vi "Send Message And Wait For Response.vi"(7 "Message Priority (Normal)":T1=enum."Normal", 8 "error in (no error)":errorcluster, 9 "timeout in ms (-1)":i32=-1, 10 "Original Message":refnum<class "Reply Msg.lvclass">, 11 "Message Enqueuer in":refnum<class "Message Enqueuer.lvclass">) -> (0 "error out":errorcluster, 1 "timed out?":bool, 2 "Reply":variant, 3 "Message Enqueuer out":refnum<class "Message Enqueuer.lvclass">)   [LabVIEW 2020, in "Reply Msg.lvclass"]
doc: "This message is <b>DEPRECATED</b>. Please replace it with <b>AF Specialty Messages.lvlib:Reply Msg.lvclass</b>, which provides the same functionality and a cleaner PPL build experience.\n\n<p>(<strong>Filename</strong>: <span class=\"dnl\">Actor Framework.lvlib:Reply Msg.lvclass:Send Message And Wait For Response.vi</span>)</p>\n\n<p>Sends a message to an actor and synchronously waits for a response from the actor.</p>"
uses:
  Reply Msg.lvclass
  C:/dev/actor-framework/dist/vi.lib/ActorFramework/Message/Message.lvclass
  Message Enqueuer/Message Enqueuer.lvclass
  Reply Msg.lvclass/Reply Msg.ctl
  Message Enqueuer/Message Enqueuer.lvclass/Message Enqueuer.ctl
  Message Enqueuer/Message Priority.ctl
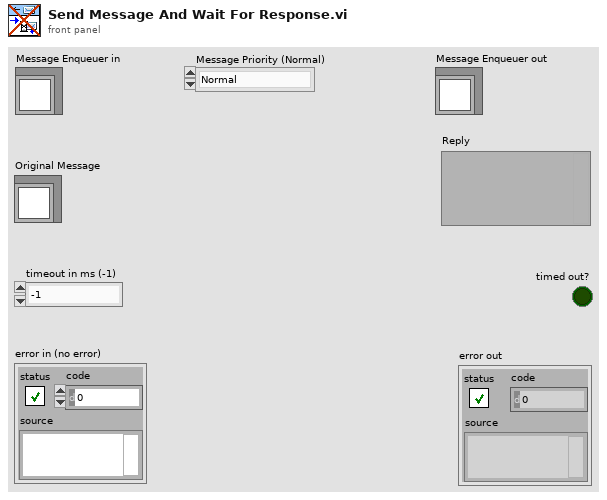
[diagram p1: front panel]
types:
  T1 = typedef "Actor Framework.lvlib/Message Enqueuer.lvclass/Message Priority.ctl" = enum16{"Low", "Normal", "High"}
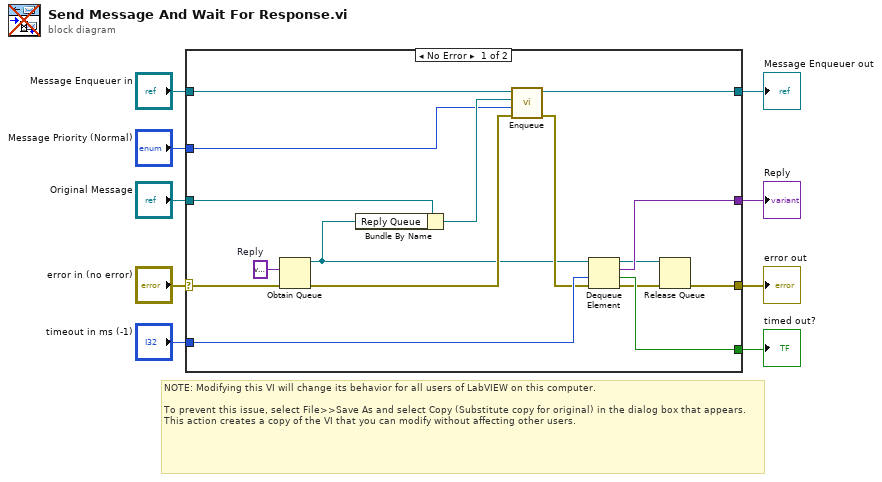
[diagram p0: block diagram]
diagram:
  # "NOTE: Modifying this VI will change its behavior for all users of LabVIEW on this computer.\n\nTo prevent this issue, select File>>Save As and select Copy (Substitute copy for original) in the dialog box that appears. This action creates a copy of the VI that you can modify without affecting other users."
  n1 = case shown="No Error" "error in (no error)" {
    selector: "error in (no error)" -> [w24 w27]
    tunnel: [w18 w27] -> w8
    tunnel: "Original Message" -> [w25 _]
    tunnel: "Message Enqueuer in" -> [w17 w26]
    tunnel: [w23 _] -> w2
    tunnel: "timeout in ms (-1)" -> [w22 _]
    tunnel: [w21 _] -> w5
    tunnel: "Message Priority (Normal)" -> [w12 _]
    tunnel: [w10 w26] -> w1
    frame No Error {
      w11 = variant  # Reply
      n2 = Obtain Queue(element data type=w11, error in (no error)=w24) -> (queue out=w13:refnum<queue>, error out=w15:errorcluster)  [unwired: 3 in, 1 out]
      n3 = Bundle By Name(cluster=w25, "Reply Queue"=w13) -> (w16:refnum<class "Reply Msg.lvclass">)
      n4 = call "Enqueue.vi"("error in (no error)"=w15, "Message Priority (Normal)"=w12, "Message"=w16, "Message Enqueuer in"=w17) -> ("error out"=w14:errorcluster, "Message Enqueuer out"=w10:refnum<class "Message Enqueuer.lvclass">)  [unwired: 6 in]
      n5 = Dequeue Element(queue=w13, timeout in ms (-1)=w22, error in (no error)=w14) -> (queue out=w19:refnum<queue>, element=w23:variant, timed out?=w21:bool, error out=w20:errorcluster)
      n6 = Release Queue(queue=w19, error in (no error)=w20) -> (error out=w18:errorcluster)  [unwired: 1 in, 2 out]
    }
    frame Error {
    }
  }
  "error out" <- w8
  "timed out?" <- w5
  "Reply" <- w2
  "Message Enqueuer out" <- w1
